vi "camera.vi"() -> ()   [LabVIEW 2022 SP3]
uses:
  <vilib>/userdefined/High Color/IMAQdx.ctl
  <vilib>/vision/driver/NI_Vision_Acquisition_Software.lvlib
panel:
  in  "停止":bool
  in  "Session In":T1
  out "Camera":T2(plugin-control)
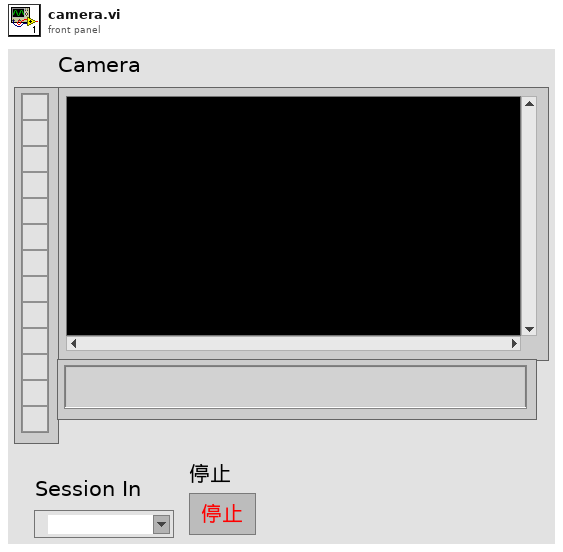
[diagram p1: front panel]
types:
  T1 = typedef "IMAQdx.ctl" = refnum<k21>
  T2 = typedef "IMAQ Image.ctl" = refnum<image>
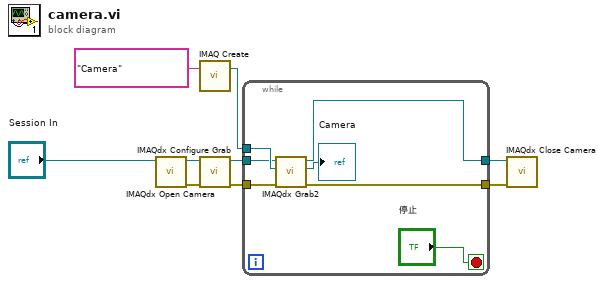
[diagram p0: block diagram]
diagram:
  n1 = call <vilib>:"IMAQdx Open Camera.vi"("Session In"="Session In") -> ("error out"=w2:errorcluster, "Session Out"=w4:T1)  [unwired: 9 in]
  n2 = call "IMAQ Create"("Image Name"="Camera") -> ("New Image"=w8:T2)  [unwired: 4 in, 1 out]
  n3 = call <vilib>:"IMAQdx Configure Grab.vi"("error in"=w2, "Session In"=w4) -> ("error out"=w1:errorcluster, "Session Out"=w3:T1)  [unwired: 8 in]
  n4 = while {
    tunnel: w8 -> [w14]
    tunnel: w1 -> [w15]
    tunnel: w3 -> [w13]
    tunnel: [w11] -> w6
    tunnel: [w10] -> w5
    stop <- "停止" stop-if-true
    n5 = call <vilib>:"IMAQdx Grab2.vi"("error in"=w15, "Image In"=w14, "Session In"=w13) -> ("error out"=w10:errorcluster, "Image Out"=→"Camera":T2, "Session Out"=w11:T1)  [unwired: 5 in, 1 out]
  }
  n6 = call <vilib>:"IMAQdx Close Camera.vi"("error in"=w5, "Session In"=w6) -> ()  [unwired: 9 in, 1 out]
